vi "readTableAsString.vi"(8 "error in (no error)":errorcluster, 11 "MS-Word in":refnum<class "MS-Word.lvclass">) -> (0 "error out":errorcluster, 2 "Table":string[][](array[string]), 3 "MS-Word out":refnum<class "MS-Word.lvclass">)   [LabVIEW 2017, in "LabVIEW NPOI.lvlib" / "MS-Word.lvclass"]
doc: "Protected dynamic dispatch method to append the wire <b>Table</b> as 2D array of strings to the <b>Document</b> as a table."
uses:
  MS-Word.lvclass
  MS-Word.lvclass/MS-Word.ctl
  xwpfDocument/xwpfDocument.lvclass/xwpfDocument.ctl
  xwpfDocument/Get Elements.Text.vi
  xwpfDocument.Element/xwpfDocument.Element.lvclass
  xwpfDocument/xwpfDocument.lvclass
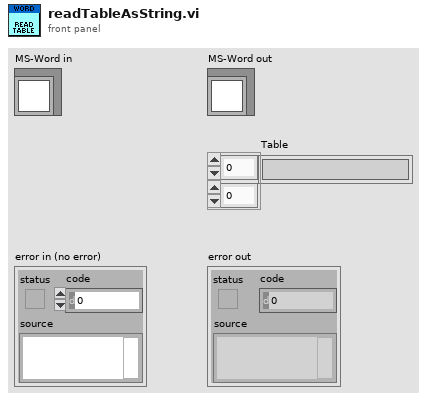
[diagram p1: front panel]
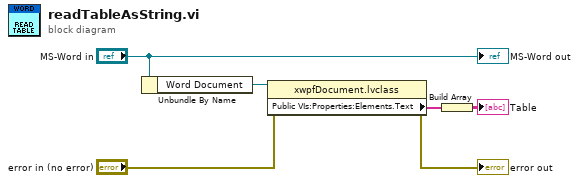
[diagram p0: block diagram]
diagram:
  n1 = Unbundle By Name("MS-Word in") -> ("Word Document"=w5:refnum<class "xwpfDocument.lvclass">)
  n2 = property class="xwpfDocument.lvclass"(reference=w5, error in="error in (no error)") -> (error out=→"error out":errorcluster, "Public VIs:Properties:Elements.Text"=w4:string[])  [unwired: 1 out]
  n3 = Build Array(w4) -> (→"Table":string[][])
  "MS-Word out" <- "MS-Word in"
